vi "Core Action.vi"(8 "error in (no error)":errorcluster, 10 "SECS-II Class":refnum<class "SECS-II Class.lvclass">, 11 "17-Deleting a Process Program by Host in":refnum<class "17-Deleting a Process Program by Host.lvclass">) -> (0 "error out":errorcluster, 2 "SECS-II Class Out":refnum<class "SECS-II Class.lvclass">, 3 "17-Deleting a Process Program by Host out":refnum<class "17-Deleting a Process Program by Host.lvclass">)   [LabVIEW 2020, in "SECS Scenarios.lvlib" / "17-Deleting a Process Program by Host.lvclass"]
uses:
  17-Deleting a Process Program by Host.lvclass
  D:/Dropbox/SECS/SECS_GEM v1.1.0/Com/SECS Scenarios/Scenarios Class/Scenarios Class.lvclass
  SECS Communication/SECS-II Class/SECS-II Class.lvclass
  SECS Communication/S7 Message Class/S7 Message Class.lvclass
  D:/Dropbox/SECS/SECS_GEM v1.1.0/Com/SECS Communication/SECS-II Class/SECS-II Class.lvclass
  Scenarios Class/Reply State.ctl
  Scenarios Class/Scenarios Class.lvclass/Scenarios Class.ctl
  Scenarios Class/Write Reply State.vi
  Scenarios Class/Read HSMS Class.vi
  SECS Communication/HSMS Class/HSMS Class.lvclass
  Scenarios Class/Scenarios Class.lvclass
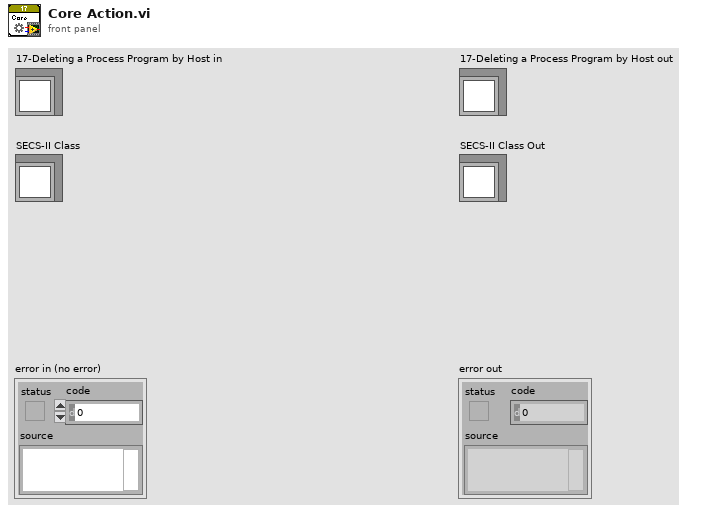
[diagram p1: front panel]
types:
  T1 = typedef "SECS Scenarios.lvlib/Scenarios Class.lvclass/Reply State.ctl" = enum16{"OK", "Illegal Data", "Unknown Stream", "Unknown Function", "Off-Line", "T3 Timeout", "Inner-Timeout"}
  T2 = typedef "SECS Communication.lvlib/S7 Message Class.lvclass/S7F18.ctl" = enum8{"Accepted", "Permission not granted", "length error", "matrix overflow", "PPID not found", "unsupported mode", "initiated for asynchronous completion", "storage limit error"}
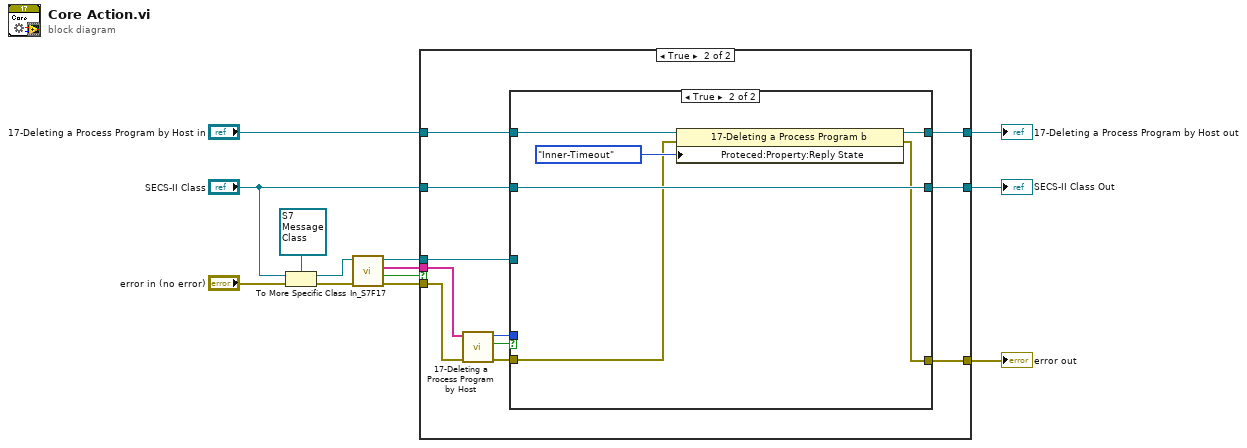
[diagram p0: block diagram]
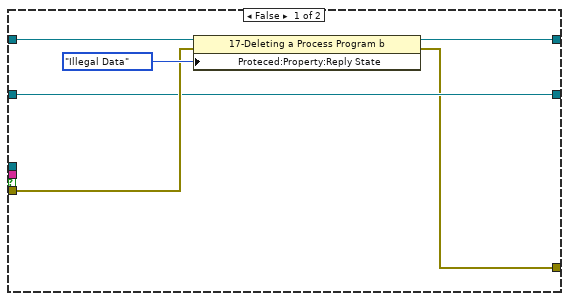
[diagram p2: hidden frame]
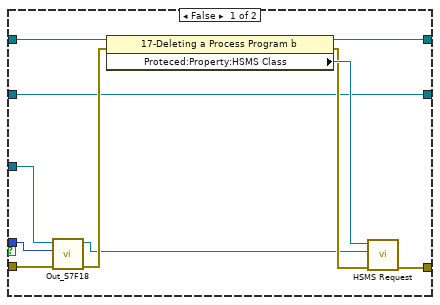
[diagram p3: hidden frame]
diagram:
  n1 = To More Specific Class(target class=refnum<class "S7 Message Class.lvclass"> refnum ("S7 Message Class in"), reference="SECS-II Class", error in="error in (no error)") -> (specific class reference=w11:refnum<class "S7 Message Class.lvclass">, error out=w12:errorcluster)
  n2 = call "In_S7F17.vi"("error in (no error)"=w12, "S7 Message Class in"=w11) -> ("error out"=w10:errorcluster, "OK?"=w1:bool, "PPID"=w6:string[], "S7 Message Class out"=w9:refnum<class "S7 Message Class.lvclass">)  [unwired: 6 in]
  n3 = case shown="True" w1 {
    tunnel: w10 -> [w17 w30]
    tunnel: w9 -> [_ w26]
    tunnel: "17-Deleting a Process Program by Host in" -> [w19 w25]
    tunnel: w6 -> [_ w24]
    tunnel: [w14 w23] -> w5
    tunnel: [w16 w22] -> w4
    tunnel: "SECS-II Class" -> [w15 w21]
    tunnel: [w15 w20] -> w2
    frame False {
      n4 = property class="17-Deleting a Process Program b"(reference=w19, error in=w17, "Proteced:Property:Reply State"=Reply_State."Illegal Data" ("Reply State")) -> (reference out=w16:refnum<class "17-Deleting a Process Program by Host.lvclass">, error out=w14:errorcluster)
    }
    frame True {
      n5 = call "17-Deleting a Process Program by Host.vi"("error in (no error)"=w30, "PPID"=w24) -> ("error out"=w29:errorcluster, "Timeout?"=w28:bool, "S7F18"=w27:T2)  [unwired: 7 in]
      n6 = case shown="True" w28 {
        tunnel: w25 -> [w41 w45]
        tunnel: w26 -> [w35 _]
        tunnel: [w38 w42] -> w23
        tunnel: [w37 w43] -> w22
        tunnel: w29 -> [w36 w44]
        tunnel: w27 -> [w32 _]
        tunnel: w21 -> [w31 w47]
        tunnel: [w31 w47] -> w20
        frame False {
          n7 = call "Out_S7F18.vi"("error in (no error)"=w36, "S7F18"=w32, "S7 Message Class in"=w35) -> ("error out"=w34:errorcluster, "S7 Message Class out"=w33:refnum<class "S7 Message Class.lvclass">)  [unwired: 7 in]
          n8 = property class="17-Deleting a Process Program b"(reference=w41, error in=w34) -> (reference out=w37:refnum<class "17-Deleting a Process Program by Host.lvclass">, error out=w39:errorcluster, "Proteced:Property:HSMS Class"=w40:refnum<class "HSMS Class.lvclass">)
          n9 = call "HSMS Request.vi"("error in (no error)"=w39, "SECS-II Class In"=w33, "HSMS Class in"=w40) -> ("error out"=w38:errorcluster)  [unwired: 7 in, 1 out]
        }
        frame True {
          n10 = property class="17-Deleting a Process Program b"(reference=w45, error in=w44, "Proteced:Property:Reply State"=Reply_State."Inner-Timeout" ("Reply State")) -> (reference out=w43:refnum<class "17-Deleting a Process Program by Host.lvclass">, error out=w42:errorcluster)
        }
      }
    }
  }
  "error out" <- w5
  "17-Deleting a Process Program by Host out" <- w4
  "SECS-II Class Out" <- w2
